vi "Sandbox.vi"(8 "error in":errorcluster) -> (0 "error out":errorcluster)   [LabVIEW 2021]
doc: "Sandbox"
uses:
  C:/Users/Petru/Documents/LabVIEW Data/PopupMenus/edit time panel and diagram/Templates/Target Library/Owned VI.vi
  C:/Users/Petru/Documents/LabVIEW Data/PopupMenus/edit time panel and diagram/Templates/Target Library/Target Library.lvlib
  <vilib>/LabVIEW Icon API/LabVIEW Icon API.lvlib
  <vilib>/LabVIEW Icon API/lv_icon/Classes/Icon/Icon.lvclass
  <vilib>/picture/picture.llb/imagedata.ctl
panel:
  out "Picture":picture
  out "Color Image":T1
  out "Icon":refnum<class "Icon.lvclass">
  out "New VI Filepath":path
  out "Random Filename":string
  out "NaN/Path/Refnum?":bool
  # "Development\ncontrols/indicators useful for development and testing, but which are not outputs of the VI"
  # "Input\nInputs to the VI"
  # "Output\nOutputs of the VI"
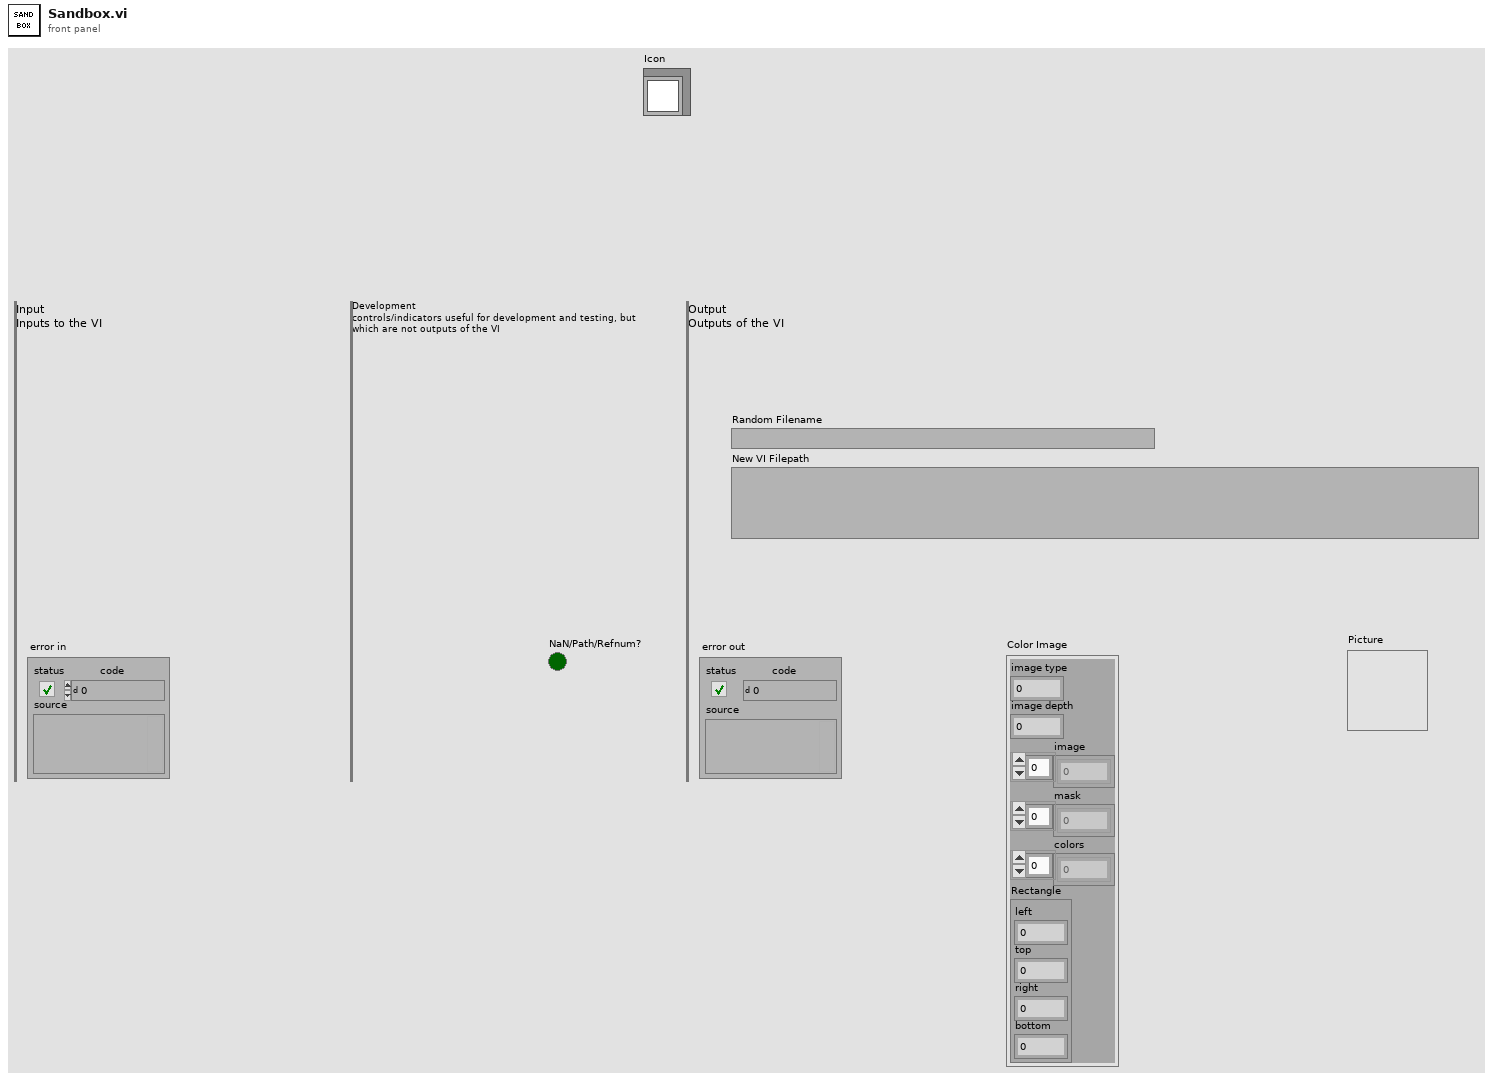
[diagram p1: front panel]
types:
  T1 = typedef "imagedata.ctl" = cluster{"image type":i32, "image depth":i32, "image":u8[], "mask":u8[], "colors":u32[], "Rectangle":cluster{"left":i16, "top":i16, "right":i16, "bottom":i16}}
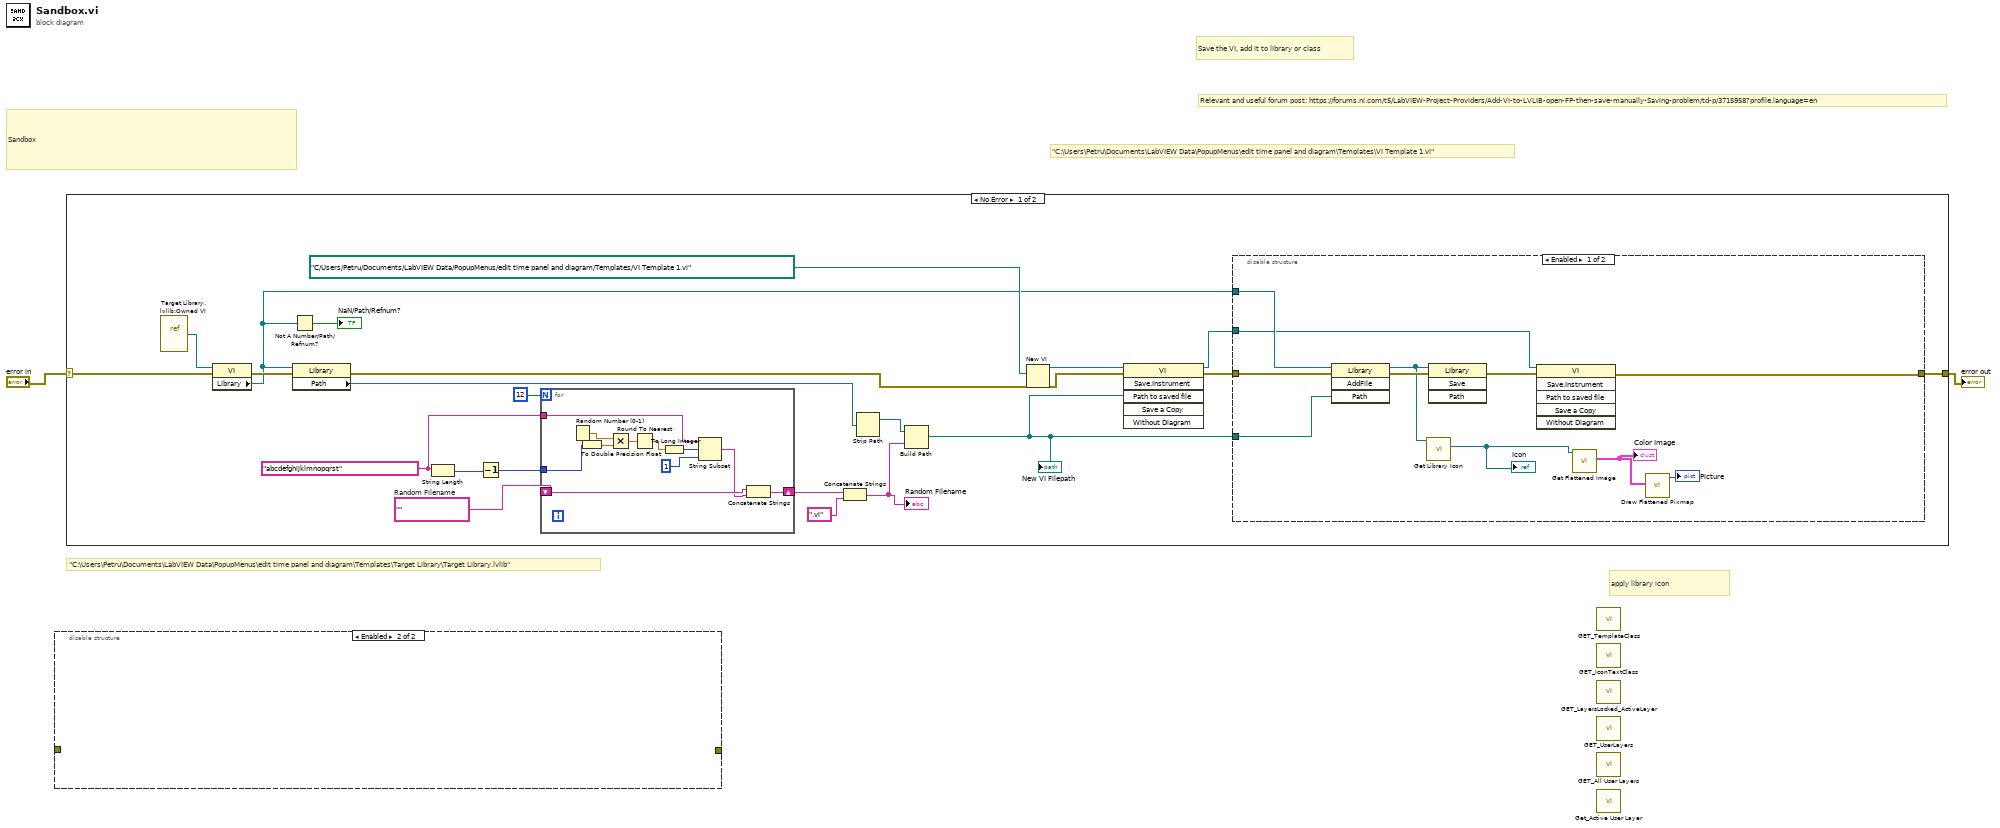
[diagram p0: block diagram]
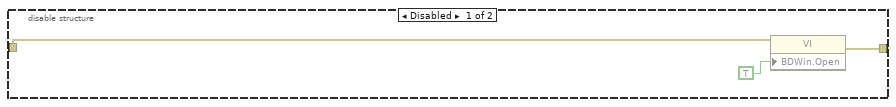
[diagram p2: hidden frame]
diagram:
  # "apply library icon"
  # "Relevant and useful forum post: https://forums.ni.com/t5/LabVIEW-Project-Providers/Add-VI-to-LVLIB-open-FP-then-save-manually-Saving-problem/td-p/3715958?profile.language=en"
  # "Save the VI, add it to library or class"
  # "\"C:\\Users\\Petru\\Documents\\LabVIEW Data\\PopupMenus\\edit time panel and diagram\\Templates\\Target Library\\Target Library.lvlib\""
  # "\"C:\\Users\\Petru\\Documents\\LabVIEW Data\\PopupMenus\\edit time panel and diagram\\Templates\\VI Template 1.vi\""
  # "Sandbox"
  n1 = disable-structure shown="Enabled" {
    disable-tunnel: [w4 _] -> _
    disable-tunnel: _ -> [w3 _]
    frame Disabled {
      n2 = property class="VI"(error in=w3, "BDWin.Open"=TRUE ("Block Diagram Window:Open")) -> (error out=w4:errorcluster)  [unwired: 1 in, 1 out]
    }
    frame Enabled {
    }
  }
  n3 = case shown="No Error" "error in" {
    selector: "error in" -> [w28 w52]
    tunnel: [w25 w52] -> w1
    frame No Error {
      w16 = ""  # Random Filename
      w18 = "abcdefghijklmnopqrst"
      n4 = vi-ref "Target Library.lvlib:Owned VI.vi"() -> (w27:refnum<vi>)
      n5 = property class="VI"(reference=w27, error in=w28) -> (error out=w24:errorcluster, "Library"=w13:refnum<vi>)  [unwired: 1 out]
      n6 = property class="Library"(reference=w13, error in=w24) -> (error out=w14:errorcluster, "Path"=w12:path)  [unwired: 1 out]
      n7 = Not A Number/Path/Refnum?(number/path/refnum=w13) -> (NaN/Path/Refnum?=→"NaN/Path/Refnum?":bool)
      n8 = String Length(string=w18) -> (length=w20:i32)
      n9 = Decrement(x=w20) -> (x-1=w19:i32)
      n10 = for {
        N: 12 -> [_]
        tunnel: w19 -> [w49]
        tunnel: w18 -> [w47]
        shift-right: [w43] -> w10
        shift-left: w16 -> [w42]
        n11 = Random Number (0-1)() -> (number: 0 to 1=w51:dbl)
        n12 = To Double Precision Float(number=w49) -> (double precision float=w48:dbl)
        n13 = Multiply(x=w51, y=w48) -> (x*y=w50:dbl)
        n14 = Round To Nearest(number=w50) -> (nearest integer value=w45:dbl)
        n15 = To Long Integer(number=w45) -> (32bit integer=w44:i32)
        n16 = String Subset(string=w47, offset (0)=w44, length (rest)=1 ("length (rest)")) -> (substring=w41:string)
        n17 = Concatenate Strings(w42, w41) -> (w43:string)
      }
      n18 = Concatenate Strings(w10, ".vi") -> (w9:string)
      "Random Filename" <- w9
      n19 = Strip Path(path=w12) -> (stripped path=w11:path)  [unwired: 1 out]
      n20 = Build Path(base path=w11, name or relative path=w9) -> (appended path=w7:path)
      "New VI Filepath" <- w7
      n21 = New VI(8:w14, 10:path "C:/Users/Petru/Documents/LabVIEW Data/PopupMenus/edit time panel and diagram/Templates/VI Template 1.vi") -> (0:w23:errorcluster, 3:w21:refnum<vi>)  [unwired: 5 in]
      n22 = invoke class="VI" method="Save.Instrument"(reference=w21, error in=w23, "Path to saved file"=w7) -> (reference out=w6:refnum<vi>, error out=w22:errorcluster)  [unwired: 3 in, 4 out]
      n23 = disable-structure shown="Enabled" {
        disable-tunnel: [w33 w40] -> w25
        disable-tunnel: w22 -> [w38 w40]
        disable-tunnel: w13 -> [w37 _]
        disable-tunnel: w7 -> [w36 _]
        disable-tunnel: w6 -> [w34 _]
        frame Enabled {
          n24 = invoke class="Library" method="AddFile"(reference=w37, error in=w38, "Path"=w36) -> (reference out=w32:refnum<vi>, error out=w39:errorcluster)  [unwired: 1 in, 2 out]
          n25 = call <vilib>:"Get Library Icon.vi"("Library Refnum in"=w32) -> ("Icon"=w29:refnum<class "Icon.lvclass">)  [unwired: 8 in, 2 out]
          "Icon" <- w29
          n26 = invoke class="Library" method="Save"(reference=w32, error in=w39) -> (error out=w35:errorcluster)  [unwired: 2 in, 3 out]
          n27 = invoke class="VI" method="Save.Instrument"(reference=w34, error in=w35) -> (error out=w33:errorcluster)  [unwired: 4 in, 5 out]
          n28 = call <vilib>:"Get Flattened Image.vi"("lv_icon.lvlib:Icon.lvclass in"=w29) -> ("Color Image"=w30:T1)  [unwired: 7 in, 3 out]
          "Color Image" <- w30
          n29 = call <vilib>:"Draw Flattened Pixmap.vi"("image data"=w30) -> ("new picture"=→"Picture":picture)  [unwired: 8 in]
        }
        frame Disabled {
        }
      }
    }
    frame Error {
    }
  }
  "error out" <- w1
  n30 = call-dynamic "GET_TemplateClass.vi"() -> ()  [unwired: 9 in, 3 out]
  n31 = call-dynamic "GET_IconTextClass.vi"() -> ()  [unwired: 9 in, 3 out]
  n32 = call-dynamic "GET_LayersLocked_ActiveLayer.vi"() -> ()  [unwired: 8 in, 4 out]
  n33 = call-dynamic "GET_UserLayers.vi"() -> ()  [unwired: 6 in, 6 out]
  n34 = call-dynamic "GET_All User Layers.vi"() -> ()  [unwired: 9 in, 3 out]
  n35 = call-dynamic "Get_Active User Layer.vi"() -> ()  [unwired: 9 in, 3 out]
